vi "Get TimeStamp Formatted.vi"(8 "error in (no error)":errorcluster, 11 "Child_2_Class in":refnum<class "Console_Class.lvclass">) -> (0 "error out":errorcluster, 1 "TimeStamp Formatted":string, 3 "Child_2_Class out":refnum<class "Console_Class.lvclass">)   [LabVIEW 2023, in "Console_Actor.lvlib" / "Console_Class.lvclass"]
uses:
  Console_Class.lvclass
  Abstraction_Interface_Class/Abstraction_Interface_Class.lvclass
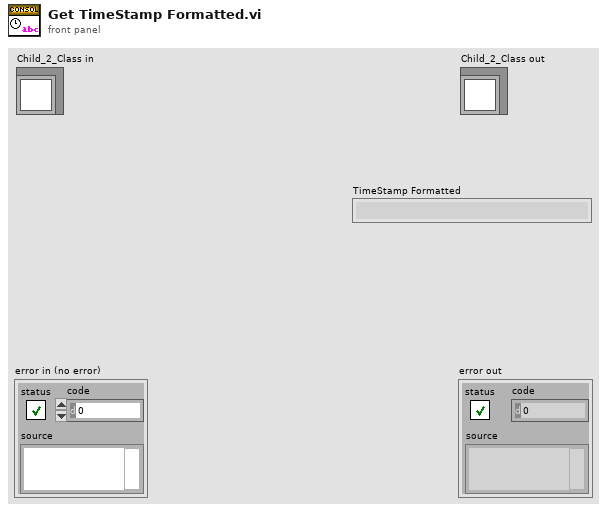
[diagram p1: front panel]
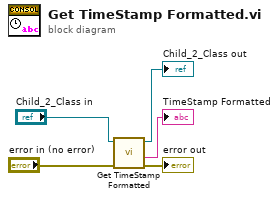
[diagram p0: block diagram]
diagram:
  n1 = call-parent "Get TimeStamp Formatted.vi"("error in (no error)"="error in (no error)", "Interface_Class in"="Child_2_Class in") -> ("error out"=→"error out":errorcluster, "TimeStamp Formatted"=→"TimeStamp Formatted":string, "Interface_Class out"=→"Child_2_Class out":refnum<class "Console_Class.lvclass">)  [unwired: 7 in]
